vi "Pad-And-Convert.vi"(11 "Array in":u8[](array[numeric])=[16, 1, 10, 0, 1, 100, 137, 240, 0, 0, 0, 0, 0, 0, 0, 0, 0] format="%.0x") -> (3 "Array":u32[](array[numeric])=[0, 268503552, 23366128, 0, 0] format="%.0x")   [LabVIEW 2018]
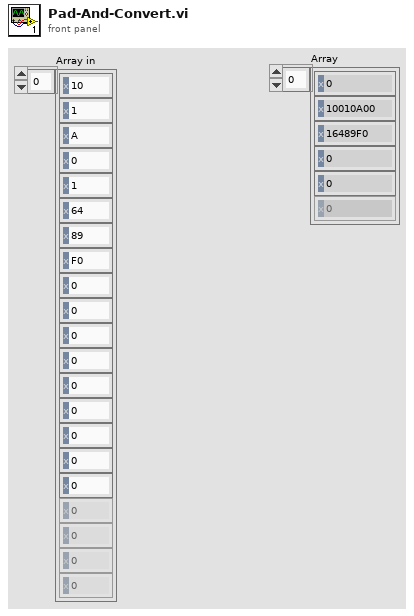
[diagram p1: front panel]
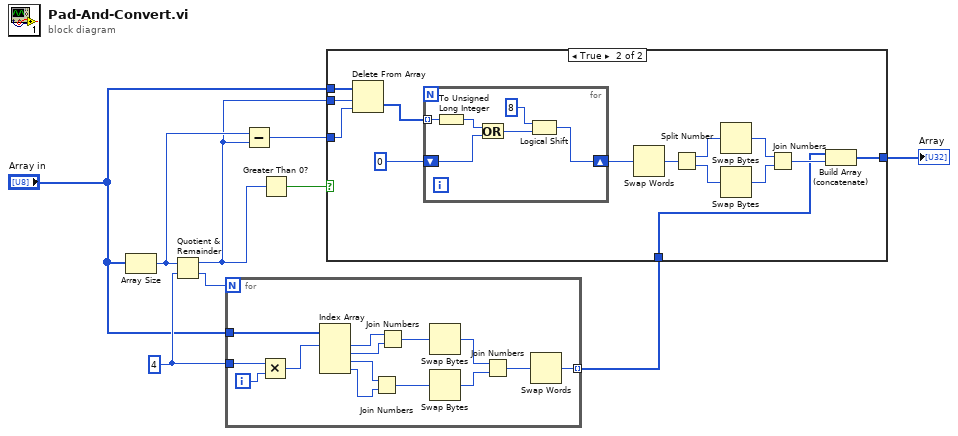
[diagram p0: block diagram]
diagram:
  w8 = 4 ("y")
  n1 = Array Size(array="Array in") -> (size(s)=w4:i32)
  n2 = Quotient & Remainder(x=w4, y=w8) -> (x-y*floor(x/y)=w3:i32, floor(x/y)=w9:i32)
  n3 = for {
    N: w9 -> [_]
    tunnel: w8 -> [w22]
    tunnel: "Array in" -> [w21]
    tunnel: [w10] -> w7 mode=indexing
    i -> [w23]
    n4 = Multiply(x=w22, y=w23) -> (x*y=w20:i32)
    n5 = Index Array(array=w21, index #1=w20) -> (element #1=w19:u8, element #2=w16:u8, element #3=w17:u8, element #4=w18:u8)  [unwired: 3 in]
    n6 = Join Numbers(hi=w17, lo=w18) -> ((hi.lo)=w12:u16)
    n7 = Join Numbers(hi=w19, lo=w16) -> ((hi.lo)=w14:u16)
    n8 = Swap Bytes(anything=w14) -> (byte swapped=w13:u16)
    n9 = Swap Bytes(anything=w12) -> (byte swapped=w11:u16)
    n10 = Join Numbers(hi=w13, lo=w11) -> ((hi.lo)=w15:u32)
    n11 = Swap Words(1:w15) -> (0:w10:u32)
  }
  n12 = Subtract(x=w4, y=w3) -> (x-y=w5:i32)
  n13 = Greater Than 0?(x=w3) -> (x > 0?=w1:bool)
  n14 = case shown="True" w1 {
    tunnel: w7 -> [w24 w25]
    tunnel: [w24 w38] -> w6
    tunnel: w5 -> [_ w37]
    tunnel: w3 -> [_ w36]
    tunnel: "Array in" -> [_ w35]
    frame False {
    }
    frame True {
      n15 = Delete From Array(array=w35, length=w36, index=w37) -> (deleted portion=w33:u8[])  [unwired: 1 out]
      n16 = for {
        shift-right: [w40] -> w32
        shift-left: u32 0 ("y") -> [w43]
        tunnel: w33 -> [w44] mode=indexing
        n17 = To Unsigned Long Integer(number=w44) -> (unsigned 32bit integer=w39:u32)
        n18 = Or(x=w39, y=w43) -> (x .or. y?=w42:u32)
        n19 = Logical Shift(y=i16 8, x=w42) -> (x << y=w40:u32)
      }
      n20 = Swap Words(1:w32) -> (0:w31:u32)
      n21 = Split Number(x=w31) -> (hi(x)=w28:u16, lo(x)=w29:u16)
      n22 = Swap Bytes(anything=w28) -> (byte swapped=w27:u16)
      n23 = Swap Bytes(anything=w29) -> (byte swapped=w26:u16)
      n24 = Join Numbers(hi=w27, lo=w26) -> ((hi.lo)=w30:u32)
      n25 = Build Array (concatenate)(w25, w30) -> (w38:u32[])
    }
  }
  "Array" <- w6
